vi "Write Display.vi"(4 "D3":u16 format="0x%04x", 5 "D0":u16 format="0x%04x", 6 "D2":u16 format="0x%04x", 7 "D1":u16 format="0x%04x", 8 "error in (no error)":errorcluster) -> (0 "error out":errorcluster)   [LabVIEW 2015]
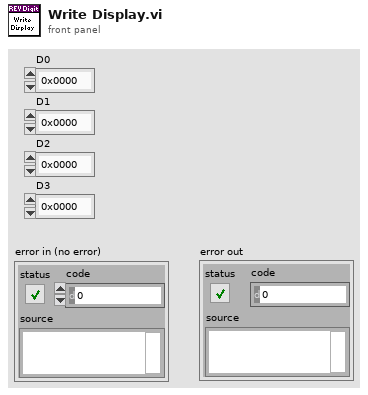
[diagram p1: front panel]
types:
  T1 = typedef "WPI_I2CDevRef.ctl" = cluster{"DevStatus":errorcluster, "Device Address":u8, "Handle":i32, "I2C Bus":T2}
  T2 = typedef "i2c_bus.ctl" = enum16{"I2C On-Board", "I2C MXP", "Invalid"}
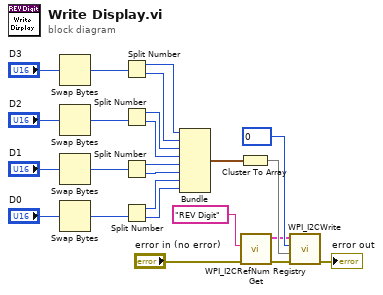
[diagram p0: block diagram]
diagram:
  n1 = Swap Bytes(anything="D3") -> (byte swapped=w4:u16)
  n2 = Swap Bytes(anything="D2") -> (byte swapped=w3:u16)
  n3 = Swap Bytes(anything="D1") -> (byte swapped=w2:u16)
  n4 = Swap Bytes(anything="D0") -> (byte swapped=w1:u16)
  n5 = Split Number(x=w4) -> (hi(x)=w16:u8, lo(x)=w17:u8)
  n6 = Split Number(x=w3) -> (hi(x)=w18:u8, lo(x)=w19:u8)
  n7 = Split Number(x=w2) -> (hi(x)=w20:u8, lo(x)=w21:u8)
  n8 = Split Number(x=w1) -> (hi(x)=w22:u8, lo(x)=w23:u8)
  n9 = Bundle(w16, w17, w18, w19, w20, w21, w22, w23) -> (w24:cluster{u8, u8, u8, u8, u8, u8, u8, u8})  [unwired: 1 in]
  n10 = Cluster To Array(cluster=w24) -> (array=w15:u8[])
  n11 = call <vilib>:"WPI_I2CRefNum Registry Get.vi"("error in (no error)"="error in (no error)", "refnum name"="REV Digit") -> ("error out"=w13:errorcluster, "I2CDevRef"=w12:T1)  [unwired: 8 in]
  n12 = call <vilib>:"WPI_I2CWrite.vi"("error in (no error)"=w13, "I2CDataToSend"=w15, "I2CRegister"=u8 0 ("Device Address"), "I2CDevRef"=w12) -> ("error out"=→"error out":errorcluster)  [unwired: 6 in, 1 out]
